vi "intepret.vi"(8 "error in (no error)":errorcluster, 10 "context":string, 11 "Expression in":refnum<class "Expression.lvclass">) -> (0 "error out":errorcluster, 2 "result":bool, 3 "Expression out":refnum<class "Expression.lvclass">)   [LabVIEW 2017, in "Expression.lvclass"]
uses:
  Expression.lvclass
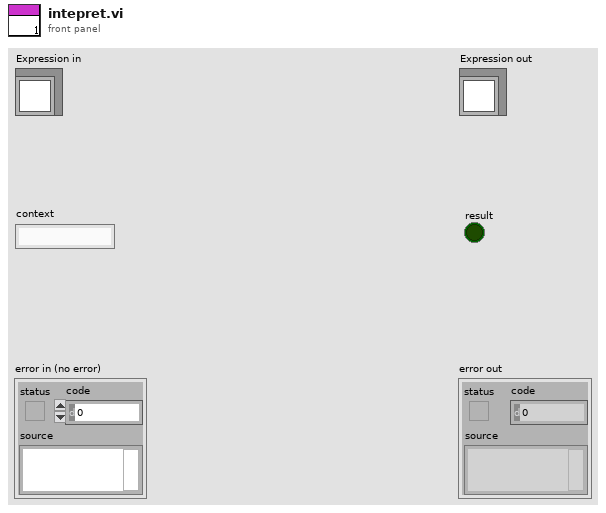
[diagram p1: front panel]
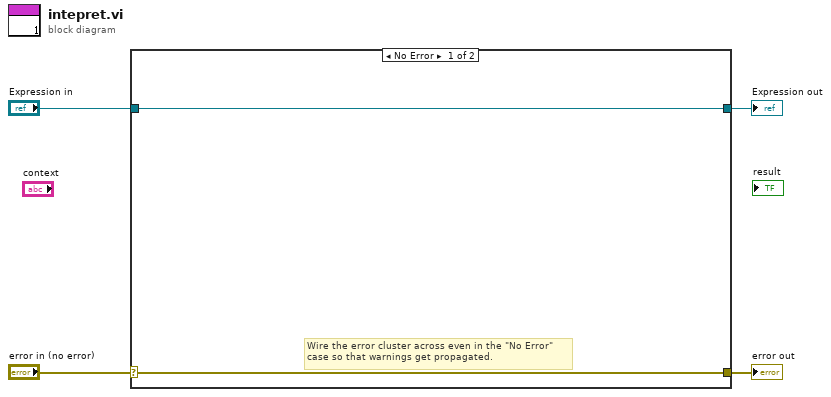
[diagram p0: block diagram]
diagram:
  n1 = case shown="No Error" "error in (no error)" {
    selector: "error in (no error)" -> [w5 w8]
    tunnel: [w5 w8] -> w3
    tunnel: [w6 w7] -> w1
    tunnel: "Expression in" -> [w6 w7]
    frame No Error {
      # "Wire the error cluster across even in the \"No Error\"\ncase so that warnings get propagated."
    }
    frame Error {
    }
  }
  "error out" <- w3
  "Expression out" <- w1
